vi "StopSignal-TestMain3.vi"() -> ()   [LabVIEW 2017]
uses:
  StopSignal.lvlib
panel:
  out "timestamp #1":timestamp
  out "timestamp #2":timestamp
  out "timestamp #3":timestamp
  out "timestamp #4":timestamp
  out "reason #4":string
  out "reason #1":string
  out "reason #2":string
  out "reason #3":string
  out "current time":timestamp
  in  "stop":bool
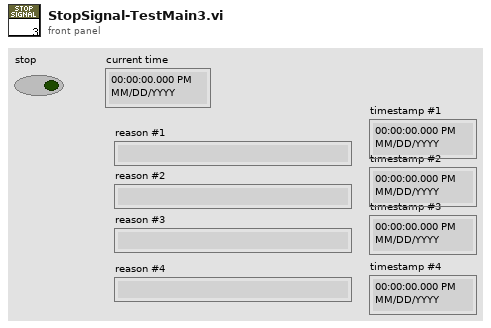
[diagram p1: front panel]
types:
  T1 = typedef "StopSignal.lvlib/StopSignal.ctl" = refnum<k1>
  T2 = typedef "StopSignal.lvlib/def-StopReason.ctl" = cluster{"Reason":string, "timestamp":timestamp}
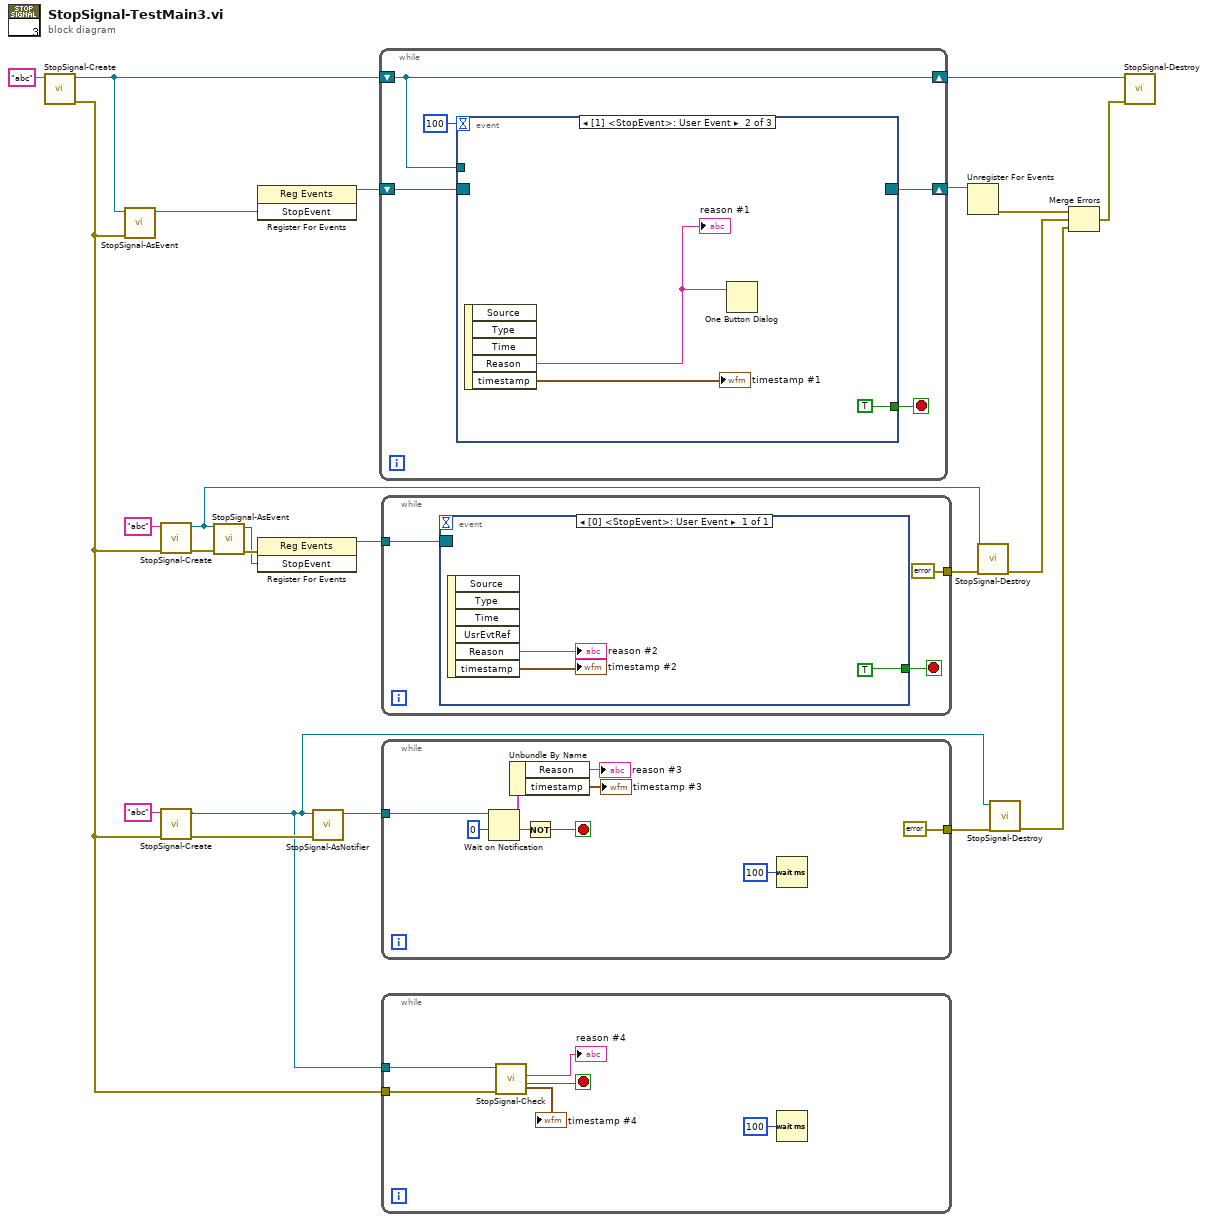
[diagram p0: block diagram]
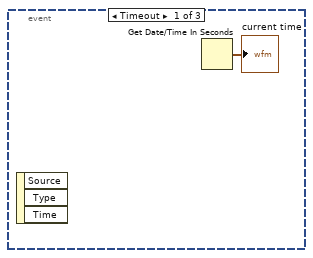
[diagram p2: hidden frame]
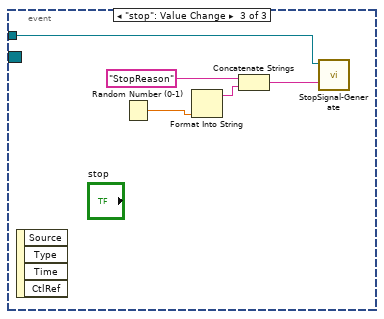
[diagram p3: hidden frame]
diagram:
  n1 = call "StopSignal-Create.vi"("name(\"\")"="abc" ("name(\"\")")) -> ("error out"=w7:errorcluster, "StopSignal"=w16:T1)  [unwired: 9 in]
  n2 = call "StopSignal-AsEvent.vi"("error in (no error)"=w7, "StopSignal"=w16) -> ("StopEvent"=w19:refnum<user-event>)  [unwired: 8 in, 1 out]
  n3 = call "StopSignal-Create.vi"("error in (no error)"=w7, "name(\"\")"="abc" ("name(\"\")")) -> ("error out"=w13:errorcluster, "StopSignal"=w10:T1)  [unwired: 8 in]
  n4 = call "StopSignal-Create.vi"("error in (no error)"=w7, "name(\"\")"="abc" ("name(\"\")")) -> ("error out"=w6:errorcluster, "StopSignal"=w5:T1)  [unwired: 8 in]
  n5 = call "StopSignal-AsEvent.vi"("error in (no error)"=w13, "StopSignal"=w10) -> ("error out"=w12:errorcluster, "StopEvent"=w11:refnum<user-event>)  [unwired: 8 in]
  n6 = register-events(w19) -> (reference out=w23:refnum<event-registration>)  [unwired: 2 in, 1 out]
  n7 = register-events(error in=w12, w11) -> (reference out=w21:refnum<event-registration>)  [unwired: 1 in, 1 out]
  n8 = call "StopSignal-AsNotifier.vi"("error in (no error)"=w6, "StopSignal"=w5) -> ("StopNotifier"=w17:refnum<notifier>)  [unwired: 8 in, 1 out]
  n9 = while {
    shift-right: [w25] -> w22
    shift-left: w23 -> [w28]
    shift-right: [w24] -> w18
    shift-left: w16 -> [w24]
    stop <- w27 stop-if-true
    n10 = event shown="[1] <StopEvent>: User Event" {
      selector: w28 -> [_ _ _]
      dyn-events: [_ _ _] -> w25
      timeout: 100 -> [_ _ _]
      tunnel: [_ TRUE _] -> w27
      tunnel: w24 -> [_ _ w33]
      event Timeout {
        n11 = event-data() -> ()  [unwired: 1 in, 3 out]
        n12 = Get Date/Time In Seconds() -> (seconds since 1Jan1904=→"current time":timestamp)
      }
      event User Event {
        n13 = event-data() -> ("Reason"=w31:string, "timestamp"=→"timestamp #1":timestamp)  [unwired: 1 in, 3 out]
        "reason #1" <- w31
        n14 = One Button Dialog(message=w31) -> ()  [unwired: 1 in, 1 out]
      }
      event "stop": Value Change {
        n15 = event-data() -> ()  [unwired: 1 in, 4 out]
        n16 = Random Number (0-1)() -> (number: 0 to 1=w36:dbl)
        n17 = Format Into String(w36) -> (resulting string=w35:string)  [unwired: 3 in, 1 out]
        n18 = Concatenate Strings("StopReason" ("event data"), w35) -> (w34:string)
        n19 = call "StopSignal-Generate.vi"("reason(\"\")"=w34, "StopSignal"=w33) -> ()  [unwired: 8 in, 2 out]
      }
    }
  }
  n20 = while {
    tunnel: w21 -> [w40]
    tunnel: [errorcluster {"status"=FALSE, "code"=0, "source"=""} ("error out")] -> w9
    stop <- w39 stop-if-true
    n21 = event shown="[0] <StopEvent>: User Event" {
      selector: w40 -> [_]
      dyn-events: _ -> [_]
      timeout: _ -> [_]
      tunnel: [TRUE] -> w39
      event User Event {
        n22 = event-data() -> ("Reason"=→"reason #2":string, "timestamp"=→"timestamp #2":timestamp)  [unwired: 1 in, 4 out]
      }
    }
  }
  n23 = while {
    tunnel: w17 -> [w48]
    tunnel: [errorcluster {"status"=FALSE, "code"=0, "source"=""} ("error out")] -> w4
    stop <- w49 stop-if-true
    n24 = Wait on Notification(notifier=w48, timeout in ms (-1)=0) -> (notification=w47:T2, timed out?=w51:bool)  [unwired: 2 in, 2 out]
    n25 = Unbundle By Name(w47) -> ("Reason"=→"reason #3":string, "timestamp"=→"timestamp #3":timestamp)
    n26 = Not(x=w51) -> (.not. x?=w49:bool)
    n27 = Wait (ms)(milliseconds to wait=u32 100) -> ()  [unwired: 1 out]
  }
  n28 = while {
    tunnel: w5 -> [w57]
    tunnel: w7 -> [w56]
    stop <- w55 stop-if-true
    n29 = call "StopSignal-Check.vi"("error in (no error)"=w56, "StopSignal"=w57) -> ("Stop?"=w55:bool, "Reason"=→"reason #4":string, "timestamp"=→"timestamp #4":timestamp)  [unwired: 5 in, 2 out]
    n30 = Wait (ms)(milliseconds to wait=u32 100) -> ()  [unwired: 1 out]
  }
  n31 = Unregister For Events(event registration refnum=w22) -> (error out=w20:errorcluster)  [unwired: 1 in]
  n32 = call "StopSignal-Destroy.vi"("error in (no error)"=w9, "StopSignal"=w10) -> ("error out"=w2:errorcluster)  [unwired: 9 in]
  n33 = call "StopSignal-Destroy.vi"("error in (no error)"=w4, "StopSignal"=w5) -> ("error out"=w1:errorcluster)  [unwired: 9 in]
  n34 = Merge Errors(w20, w2, w1) -> (w3:errorcluster)
  n35 = call "StopSignal-Destroy.vi"("error in (no error)"=w3, "StopSignal"=w18) -> ()  [unwired: 9 in, 1 out]
